vi "Serial.vi"() -> (0 "semaphore error out":errorcluster, 1 "semaphore":T1, 2 "VISA error out":errorcluster, 3 "VISA out":refnum<visa-resource-name>)   [LabVIEW 2018]
panel:
  in  "Semaphore Error In (no error)":errorcluster
  in  "Timeout (5000 msec)":u32=5000
  in  "Serial Configuration":T2={"Baud Rate"=9600, "Parity"=0, "Data Bits"=8, "Stop Bits"=10, "Flow Control"=0} {"Flow Control" items=["None", "XON/XOFF", "RTS/CTS", "XON/XOFF & RTS/CTS", "DTR/DSR", "XON/XOFF & DTR/DSR"]; "Stop Bits" items=["1.0"=10, "1.5"=15, "2.0"=20]; "Data Bits" items=["7"=7, "8"=8]; "Parity" items=["None", "Odd", "Even", "Mark", "Space"]; "Baud Rate" items=["300"=300, "600"=600, "1200"=1200, "2400"=2400, "4800"=4800, "9600"=9600, "19200"=19200]}
  in  "VISA resource name":refnum<visa-resource-name>
  in  "error in (no error)":errorcluster
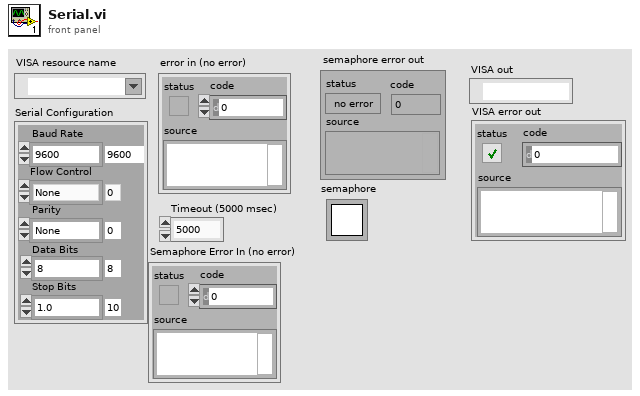
[diagram p1: front panel]
types:
  T1 = typedef "Semaphore RefNum" = refnum<k1>
  T2 = cluster{"Baud Rate":u32, "Parity":u16, "Data Bits":u16, "Stop Bits":u16, "Flow Control":u16}
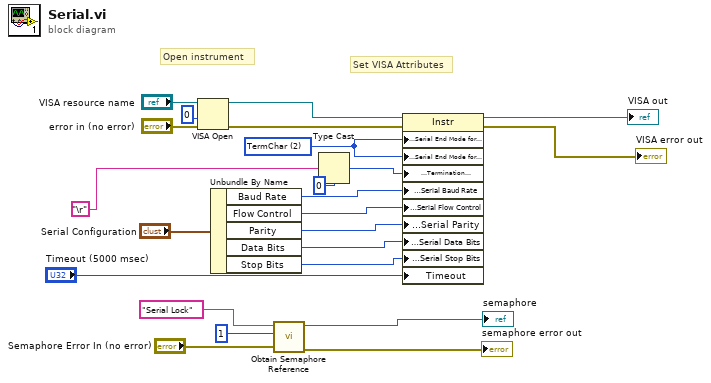
[diagram p0: block diagram]
diagram:
  w9 = u16 2 items=["None", "LastBit", "TermChar"] ("Serial Settings:Serial End Mode for Reads")
  # "Set VISA Attributes"
  # "Open instrument"
  n1 = VISA Open(access mode=u32 0, error in (no error)="error in (no error)", VISA resource name="VISA resource name") -> (VISA resource name=w12:refnum<visa-resource-name>, error out=w13:errorcluster)  [unwired: 2 in]
  n2 = Unbundle By Name("Serial Configuration") -> ("Baud Rate"=w19:u32, "Flow Control"=w15:u16, "Parity"=w17:u16, "Data Bits"=w18:u16, "Stop Bits"=w14:u16)
  n3 = call <vilib>:"Obtain Semaphore Reference.vi"("error in (no error)"="Semaphore Error In (no error)", "size (1)"=1, "name (unnamed)"="Serial Lock") -> ("error out"=→"semaphore error out":errorcluster, "semaphore"=→"semaphore":T1)  [unwired: 2 in, 1 out]
  n4 = Type Cast(type=u8 0, x="\r") -> (*(type *) &x=w11:u8)
  n5 = property class="Instr"(reference=w12, error in=w13, "Serial Settings:Serial End Mode for Reads"=w9, "Serial Settings:Serial End Mode for Writes"=w9, "Message Based Settings:Termination Character"=w11, "Serial Settings:Serial Baud Rate"=w19, "Serial Settings:Serial Flow Control"=w15, "Serial Settings:Serial Parity"=w17, "Serial Settings:Serial Data Bits"=w18, "Serial Settings:Serial Stop Bits"=w14, "Timeout"="Timeout (5000 msec)") -> (reference out=→"VISA out":refnum<visa-resource-name>, error out=→"VISA error out":errorcluster)
